vi "Lidar Finder.vi"(5 "VISA resource name":refnum<visa-resource-name>="Hukuyo") -> (0 "Objects":cluster{i32, i32}[](array[cluster]), 1 "Widest Object":cluster{i32, i32}, 2 "Where to Point":i32)   [LabVIEW 2014]
uses:
  <instrlib>/Hokuyo URG Series/Public/Initialize-Standard.vi
  <instrlib>/Hokuyo URG Series/Hokuyo URG Series.lvlib
panel:
  in  "Tab Control":enum32{"Raw Data", "Clean Data"}(tab)
  out "Data Aquired":picture
  out "Object Graph":i32[](graph)
  out "Edges":i32[](graph)
  in  "polar attributes (hidden)":T1={"maximum"=30000.0, "minimum"=0.0, "clip to min"=FALSE, "log?(F)"=TRUE, "grid color"=6710886, "plot color"=65280, "fmt and prec"={"format"=enum."Decimal", "precision"=0}, "visible section"=8} {"minimum" format="%0.2f"; "maximum" format="%0.2f"}
  in  "Grid Color":u32(colorbox)=11776947
  in  "Plot Color":u32(colorbox)=14422272
  in  "Max (m)":dbl=1.0
  in  "End Point":dbl=40.0
  in  "Start Point":dbl=-50.0
  in  "Cluster Count":dbl=1.0
  in  "Encoding Width":u16(ring)=3 items=["2 Byte"=2, "3 Byte"=3]
  # "click here to run"
  # "Hokuyo LIDAR Example"
  # "Plot in mm"
  # "start at-50"
  # "start at 40"
  # "Start with 1.0 m"
  # "Hokuyo plugged in?"
  # "Location"
  # "Width"
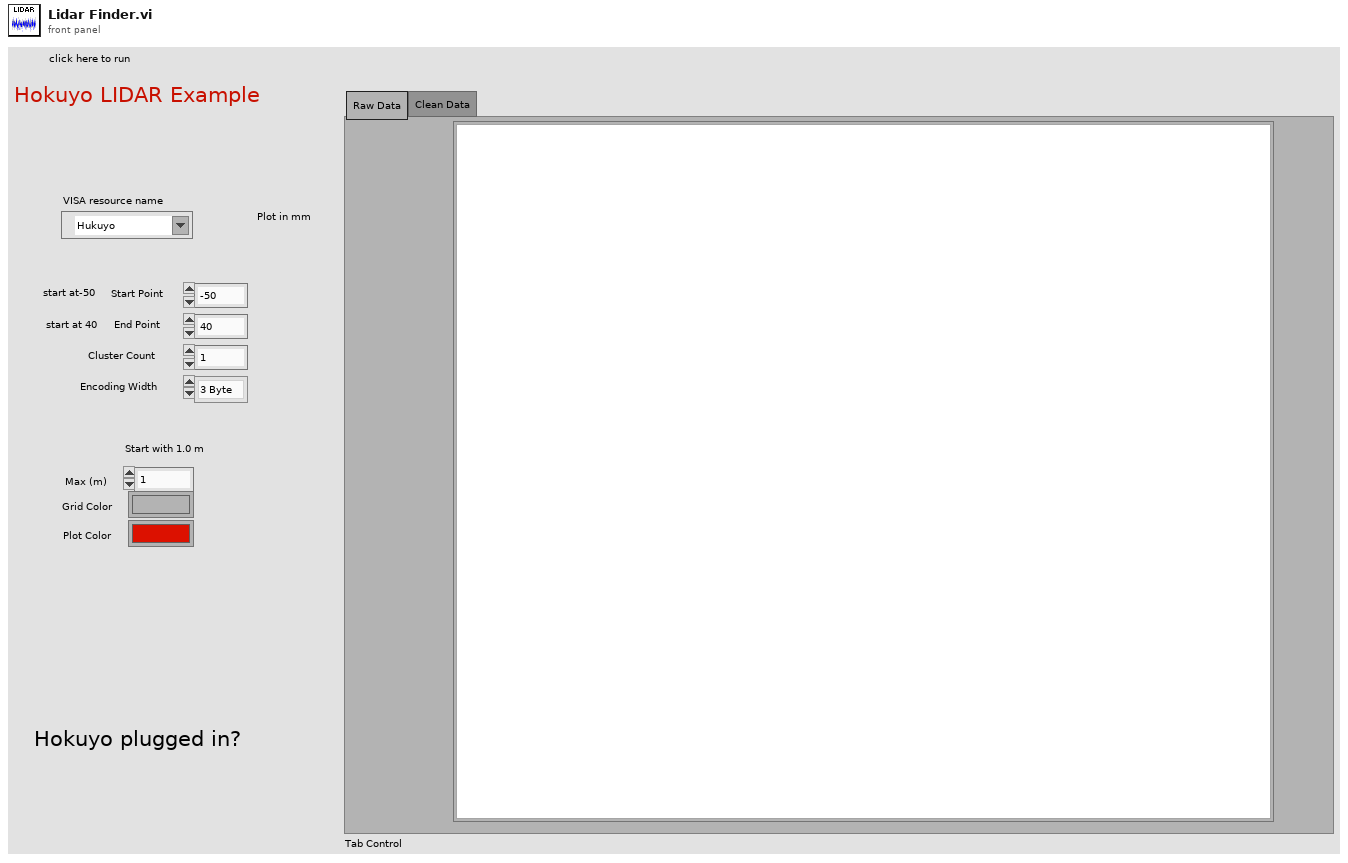
[diagram p1: front panel]
types:
  T1 = cluster{"maximum":dbl, "minimum":dbl, "clip to min":bool, "log?(F)":bool, "grid color":u32, "plot color":u32, "fmt and prec":cluster{"format":enum8{"Decimal", "Scientific", "Engineering", "Binary", "Octal", "Hex"}, "precision":u8}, "visible section":u16}
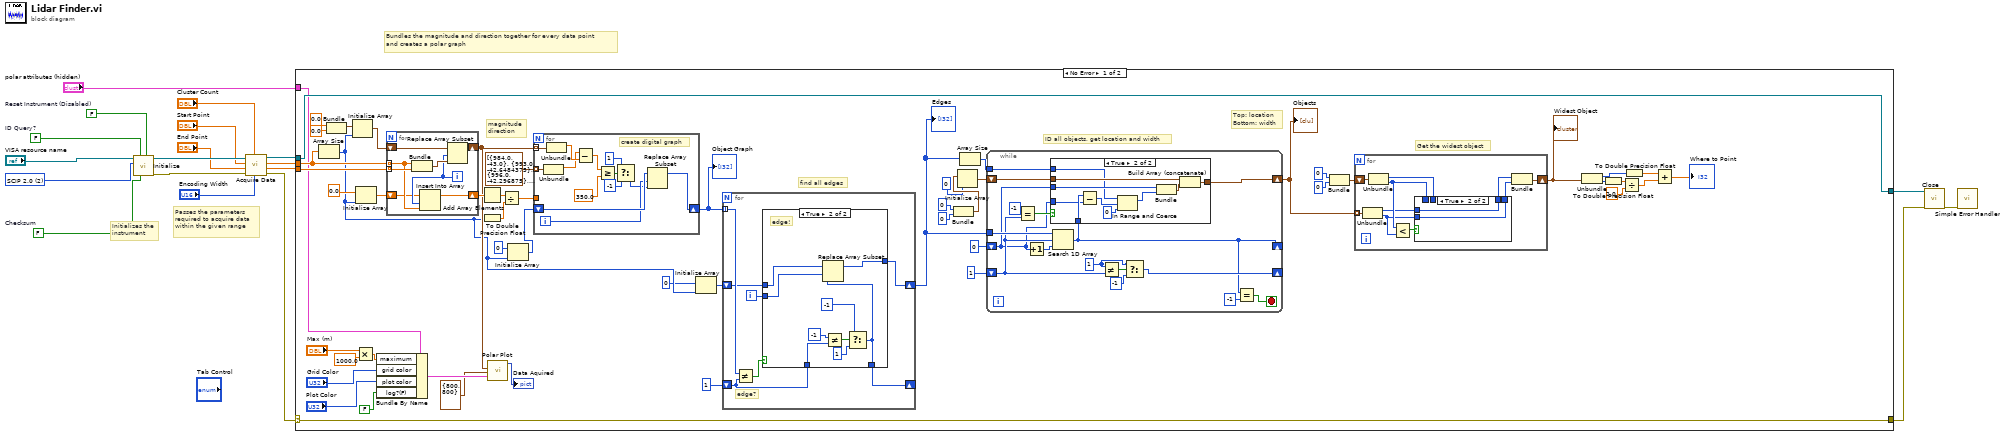
[diagram p0: block diagram]
diagram:
  w17 = FALSE  # Checksum
  w15 = FALSE  # ID Query?
  w13 = u32 2 items=["Convert to Latest", "SCIP 1.1", "SCIP 2.0"] ("Protocol")
  w14 = FALSE  # Reset Instrument (Disabled)
  # "Passes the parameters\nrequired to acquire data\nwithin the given range"
  # "Bundles the magnitude and direction together for every data point\nand creates a polar graph"
  # "Initializes the instrument"
  n1 = call-poly <instrlib>:"Initialize.vi"("Reset? (F: No)"=w14, "Checksum (Disabled)"=w17, "ID Query? (Enabled)"=w15, "Protocol (2: SCIP 2.0)"=w13, "VISA resource name"="VISA resource name") -> ("error out"=w10:errorcluster, "VISA resource name out"=w11:refnum<visa-resource-name>)  [unwired: 5 in]
  n2 = call <instrlib>:"Acquire Data.vi"("Data Encoding Width (3 Byte)"="Encoding Width", "Cluster Count (1)"="Cluster Count", "error in (no error)"=w10, "End Point (120°)"="End Point", "Start Point (-120°)"="Start Point", "VISA resource name"=w11) -> ("error out"=w5:errorcluster, "Direction"=w6:dbl[], "Magnitude"=w7:dbl[], "VISA resource name out"=w8:refnum<visa-resource-name>)  [unwired: 2 in]
  n3 = case shown="No Error" w5 {
    selector: w5 -> [w71 w155]
    tunnel: [w71 w155] -> w19
    tunnel: w8 -> [w72 w154]
    tunnel: [w72 w154] -> w12
    tunnel: w7 -> [w66 _]
    tunnel: w6 -> [w65 _]
    tunnel: "polar attributes (hidden)" -> [w63 _]
    frame No Error {
      # "Get the widest object"
      # "Top: location\nBottom: width"
      # "find all edges"
      # "ID all objects, get location and width"
      # "magnitude\ndirection"
      n4 = Array Size(array=w66) -> (size(s)=w45:i32)
      n5 = Bundle(0.0, 0.0) -> (w68:cluster{dbl, dbl})  [unwired: 1 in]
      n6 = Initialize Array(w68, w45) -> (w67:cluster{dbl, dbl}[])
      n7 = Multiply(x="Max (m)", y=1000.0) -> (x*y=w59:dbl)
      n8 = Initialize Array(0.0, w45) -> (w54:dbl[])
      n9 = Bundle By Name(cluster=w63, "maximum"=w59, "grid color"="Grid Color", "plot color"="Plot Color", "log?(F)"=FALSE) -> (w64:T1)
      n10 = for {
        shift-right: [w151] -> w50
        shift-left: w67 -> [w152]
        tunnel: w66 -> [w148] mode=indexing
        tunnel: w65 -> [w153] mode=indexing
        shift-right: [w146] -> w53
        shift-left: w54 -> [w147]
        i -> [w149]
        n11 = Bundle(w148, w153) -> (w150:cluster{dbl, dbl})  [unwired: 1 in]
        n12 = Insert Into Array(array=w147, index=w149, new element=w148) -> (w146:dbl[])
        n13 = Replace Array Subset(array=w152, new element=w150, index=w149) -> (w151:cluster{dbl, dbl}[])
      }
      n14 = Add Array Elements(numeric array=w53) -> (sum=w52:dbl)
      n15 = To Double Precision Float(number=w45) -> (double precision float=w51:dbl)
      n16 = call <vilib>:"Polar Plot.vi"("polar attributes"=w64, "dimensions (w,h)"=cluster{"width":i16, "height":i16} {"width"=800, "height"=800}, "data array [mag, phase (deg)]"=w50) -> ("new picture"=→"Data Aquired":picture)  [unwired: 8 in]
      n17 = Divide(x=w52, y=w51) -> (x/y=w49:dbl)
      n18 = Initialize Array(0, w45) -> (w48:i32[])
      n19 = for {
        tunnel: w50 -> [w145] mode=indexing
        tunnel: w49 -> [_]
        shift-right: [w142] -> w20
        shift-left: w48 -> [w144]
        tunnel: cluster{dbl, dbl}[] [{984.0, -43.0}, {993.0, -42.6484375}, {996.0, -42.296875}, {1001.0, -41.9453125}, {1013.0, -41.59375}, {1018.0, -41.2421875}, {1021.0, -40.890625}, {1026.0, -40.5390625}, {1029.0, -40.1875}, {1029.0, -39.8359375}, {1050.0, -39.484375}, {1067.0, -39.1328125}, {1067.0, -38.78125}, {1067.0, -38.4296875}, {1070.0, -38.078125}, {1088.0, -37.7265625}, {1098.0, -37.375}, {1102.0, -37.0234375}, {1107.0, -36.671875}, {1107.0, -36.3203125}, {1126.0, -35.96875}, {1127.0, -35.6171875}, {1141.0, -35.265625}, {1144.0, -34.9140625}, {1161.0, -34.5625}, {1165.0, -34.2109375}, {1187.0, -33.859375}, {1189.0, -33.5078125}, {1262.0, -33.15625}, {1263.0, -32.8046875}, {1263.0, -32.453125}, {1263.0, -32.1015625}, {1258.0, -31.75}, {1258.0, -31.3984375}, {1238.0, -31.046875}, {1187.0, -30.6953125}, {1075.0, -30.34375}, {1047.0, -29.9921875}, {1037.0, -29.640625}, {1037.0, -29.2890625}, {1046.0, -28.9375}, {1046.0, -28.5859375}, {1037.0, -28.234375}, {1017.0, -27.8828125}, {1017.0, -27.53125}, {1017.0, -27.1796875}, {1020.0, -26.828125}, {1026.0, -26.4765625}, {1030.0, -26.125}, {1035.0, -25.7734375}, {1030.0, -25.421875}, {1026.0, -25.0703125}, {1014.0, -24.71875}, {1004.0, -24.3671875}, {993.0, -24.015625}, {993.0, -23.6640625}, {993.0, -23.3125}, {998.0, -22.9609375}, {1018.0, -22.609375}, {1022.0, -22.2578125}, {1033.0, -21.90625}, {1035.0, -21.5546875}, {1035.0, -21.203125}, {1038.0, -20.8515625}, {1038.0, -20.5}, {1039.0, -20.1484375}, {1044.0, -19.796875}, {1044.0, -19.4453125}, {1042.0, -19.09375}, {1044.0, -18.7421875}, {1042.0, -18.390625}, {1038.0, -18.0390625}, {1038.0, -17.6875}, {1035.0, -17.3359375}, {1033.0, -16.984375}, {1028.0, -16.6328125}, {1024.0, -16.28125}, {1024.0, -15.9296875}, {1015.0, -15.578125}, {1015.0, -15.2265625}, {1013.0, -14.875}, {1013.0, -14.5234375}, {1015.0, -14.171875}, {1015.0, -13.8203125}, {1013.0, -13.46875}, {1013.0, -13.1171875}, {1010.0, -12.765625}, {1006.0, -12.4140625}, {1006.0, -12.0625}, {1004.0, -11.7109375}, {1006.0, -11.359375}, {1004.0, -11.0078125}, {1003.0, -10.65625}, {998.0, -10.3046875}, {1003.0, -9.953125}, {1003.0, -9.6015625}, {1003.0, -9.25}, {994.0, -8.8984375}, {993.0, -8.546875}, {993.0, -8.1953125}, {993.0, -7.84375}, {997.0, -7.4921875}, {997.0, -7.140625}, {997.0, -6.7890625}, {993.0, -6.4375}, {991.0, -6.0859375}, {991.0, -5.734375}, {988.0, -5.3828125}, {988.0, -5.03125}, {988.0, -4.6796875}, {988.0, -4.328125}, {986.0, -3.9765625}, {989.0, -3.625}, {989.0, -3.2734375}, {989.0, -2.921875}, {989.0, -2.5703125}, {989.0, -2.21875}, {989.0, -1.8671875}, {989.0, -1.515625}, {984.0, -1.1640625}, {982.0, -0.8125}, {982.0, -0.4609375}, {981.0, -0.109375}, {981.0, 0.2421875}, {988.0, 0.59375}, {988.0, 0.9453125}, {988.0, 1.296875}, {988.0, 1.6484375}, {985.0, 2.0}, {985.0, 2.3515625}, {985.0, 2.703125}, {985.0, 3.0546875}, {985.0, 3.40625}, {985.0, 3.7578125}, {992.0, 4.109375}, {992.0, 4.4609375}, {991.0, 4.8125}, {991.0, 5.1640625}, {991.0, 5.515625}, {991.0, 5.8671875}, {994.0, 6.21875}, {994.0, 6.5703125}, {994.0, 6.921875}, {994.0, 7.2734375}, {989.0, 7.625}, {989.0, 7.9765625}, {995.0, 8.328125}, {998.0, 8.6796875}, {999.0, 9.03125}, {1003.0, 9.3828125}, {1003.0, 9.734375}, {1003.0, 10.0859375}, {1008.0, 10.4375}, {1008.0, 10.7890625}, {1006.0, 11.140625}, {1008.0, 11.4921875}, {1006.0, 11.84375}, {1006.0, 12.1953125}, {1017.0, 12.546875}, {1017.0, 12.8984375}, {1017.0, 13.25}, {1018.0, 13.6015625}, {1018.0, 13.953125}, {1020.0, 14.3046875}, {1020.0, 14.65625}, {1020.0, 15.0078125}, {1020.0, 15.359375}, {1022.0, 15.7109375}, {1024.0, 16.0625}, {1025.0, 16.4140625}, {1034.0, 16.765625}, {1040.0, 17.1171875}, {1040.0, 17.46875}, {1040.0, 17.8203125}, {1046.0, 18.171875}, {1044.0, 18.5234375}, {1044.0, 18.875}, {1044.0, 19.2265625}, {1048.0, 19.578125}, {1049.0, 19.9296875}, {1050.0, 20.28125}, {1055.0, 20.6328125}, {1060.0, 20.984375}, {1065.0, 21.3359375}, {1066.0, 21.6875}, {1070.0, 22.0390625}, {1065.0, 22.390625}, {1065.0, 22.7421875}, {1070.0, 23.09375}, {1037.0, 23.4453125}, {1036.0, 23.796875}, {1022.0, 24.1484375}, {1037.0, 24.5}, {1015.0, 24.8515625}, {1011.0, 25.203125}, {998.0, 25.5546875}, {998.0, 25.90625}, {996.0, 26.2578125}, {995.0, 26.609375}, {995.0, 26.9609375}, {1005.0, 27.3125}, {1005.0, 27.6640625}, {1008.0, 28.015625}, {1064.0, 28.3671875}, {1104.0, 28.71875}, {1106.0, 29.0703125}, {1120.0, 29.421875}, {1128.0, 29.7734375}, {1128.0, 30.125}, {1128.0, 30.4765625}, {1136.0, 30.828125}, {1144.0, 31.1796875}, {1144.0, 31.53125}, {1144.0, 31.8828125}, {1256.0, 32.234375}, {1298.0, 32.5859375}, {1304.0, 32.9375}, {1307.0, 33.2890625}, {1322.0, 33.640625}, {1327.0, 33.9921875}, {1337.0, 34.34375}, {1347.0, 34.6953125}, {1347.0, 35.046875}, {1348.0, 35.3984375}, {1352.0, 35.75}, {1358.0, 36.1015625}, {1360.0, 36.453125}, {1367.0, 36.8046875}, {1376.0, 37.15625}, {1391.0, 37.5078125}, {1393.0, 37.859375}, {1400.0, 38.2109375}, {1403.0, 38.5625}, {1407.0, 38.9140625}, {1409.0, 39.265625}, {1412.0, 39.6171875}, {1435.0, 39.96875}, {1435.0, 40.3203125}, {1443.0, 40.671875}, {1446.0, 41.0234375}, {1447.0, 41.375}, {1474.0, 41.7265625}, {1475.0, 42.078125}, {1477.0, 42.4296875}, {1489.0, 42.78125}] -> [w137] mode=indexing
        i -> [w143]
        # "create digital graph"
        n20 = Unbundle(w137) -> (w134:dbl)  [unwired: 1 out]
        n21 = Unbundle(w145) -> (w135:dbl)  [unwired: 1 out]
        n22 = Subtract(x=w134, y=w135) -> (x-y=w136:dbl)
        n23 = Greater Or Equal?(x=w136, y=350.0) -> (x >= y?=w140:bool)
        n24 = Select(t=1, s=w140, f=-1) -> (s? t:f=w141:i32)
        n25 = Replace Array Subset(array=w144, new element=w141, index=w143) -> (w142:i32[])
      }
      "Object Graph" <- w20
      n26 = Initialize Array(0, w45) -> (w43:i32[])
      n27 = for {
        tunnel: w20 -> [w120] mode=indexing
        shift-right: [w115] -> w35
        shift-left: w43 -> [w117]
        shift-right: [w119] -> _
        shift-left: 1 -> [w118]
        i -> [w116]
        # "edge?"
        n28 = Not Equal?(x=w120, y=w118) -> (x != y?=w121:bool)
        n29 = case shown="True" w121 {
          tunnel: [w123 w128] -> w119
          tunnel: w118 -> [w123 w132]
          tunnel: w117 -> [w122 w130]
          tunnel: w116 -> [_ w129]
          tunnel: [w122 w127] -> w115
          frame False {
            # "no edge"
          }
          frame True {
            # "edge!"
            n30 = Not Equal?(x=-1, y=w132) -> (x != y?=w131:bool)
            n31 = Select(t=-1, s=w131, f=1) -> (s? t:f=w128:i32)
            n32 = Replace Array Subset(array=w130, new element=w128, index=w129) -> (w127:i32[])
          }
        }
      }
      "Edges" <- w35
      n33 = Bundle(0, 0) -> (w39:cluster{i32, i32})  [unwired: 1 in]
      n34 = Initialize Array(w39, 0) -> (w40:cluster{i32, i32}[])
      n35 = Array Size(array=w35) -> (size(s)=w34:i32)
      n36 = while {
        tunnel: w35 -> [w101]
        shift-right: [w97] -> _
        shift-left: 1 -> [w92]
        shift-right: [w94] -> _
        shift-left: 0 -> [w89]
        shift-right: [w96] -> w30
        shift-left: w40 -> [w95]
        tunnel: w34 -> [w88]
        stop <- w103 stop-if-true
        w99 = 1
        n37 = Equal?(x=-1, y=w92) -> (x = y?=w91:bool)
        n38 = Increment(x=w89) -> (x+1=w90:i32)
        n39 = Search 1D Array(1D array=w101, element=w92, start index (0)=w90) -> (index of element=w94:i32)
        n40 = case shown="True" w91 {
          tunnel: [w104 w114] -> w96
          tunnel: w95 -> [w104 w113]
          tunnel: w94 -> [_ w111]
          tunnel: w89 -> [_ w110]
          tunnel: w89 -> [_ w109]
          tunnel: w88 -> [_ w108]
          frame False {
          }
          frame True {
            n41 = Subtract(x=w111, y=w110) -> (x-y=w107:i32)
            n42 = In Range and Coerce(upper limit=w108, x=w107, lower limit=0) -> (coerced(x)=w106:i32)  [unwired: 1 out]
            n43 = Bundle(w109, w106) -> (w112:cluster{i32, i32})  [unwired: 1 in]
            n44 = Build Array (concatenate)(w113, w112) -> (w114:cluster{i32, i32}[])
          }
        }
        n45 = Not Equal?(x=w99, y=w92) -> (x != y?=w98:bool)
        n46 = Select(t=w99, s=w98, f=-1) -> (s? t:f=w97:i32)
        n47 = Equal?(x=w94, y=-1) -> (x = y?=w103:bool)
      }
      "Objects" <- w30
      n48 = Bundle(0, 0) -> (w31:cluster{i32, i32})  [unwired: 1 in]
      n49 = for {
        shift-right: [w82] -> w29
        shift-left: w31 -> [w83]
        tunnel: w30 -> [w78] mode=indexing
        n50 = Unbundle(w78) -> (w75:i32, w74:i32)
        n51 = Unbundle(w83) -> (w80:i32, w76:i32)
        n52 = Less?(x=w76, y=w74) -> (x < y?=w77:bool)
        n53 = case shown="True" w77 {
          tunnel: [w85 w87] -> w81
          tunnel: w80 -> [w85 _]
          tunnel: [w84 w86] -> w79
          tunnel: w76 -> [w84 _]
          tunnel: w75 -> [_ w87]
          tunnel: w74 -> [_ w86]
          frame False {
          }
          frame True {
          }
        }
        n54 = Bundle(w81, w79) -> (w82:cluster{i32, i32})  [unwired: 1 in]
      }
      "Widest Object" <- w29
      n55 = Unbundle(w29) -> (w23:i32, w27:i32)
      n56 = To Double Precision Float(number=w27) -> (double precision float=w26:dbl)
      n57 = Divide(x=w26, y=2.0) -> (x/y=w24:dbl)
      n58 = To Double Precision Float(number=w23) -> (double precision float=w22:dbl)
      n59 = Add(x=w22, y=w24) -> (x+y=→"Where to Point":dbl)
    }
    frame Error {
    }
  }
  n60 = call <instrlib>:"Close.vi"("error in (no error)"=w19, "VISA resource name"=w12) -> ("error out"=w16:errorcluster)  [unwired: 9 in]
  n61 = call <vilib>:"Simple Error Handler.vi"("error in (no error)"=w16) -> ()  [unwired: 4 in, 5 out]
